vi "Start all.vi"() -> ()   [LabVIEW 2020, in "MeasurementService Editor.lvlib"]
uses:
  _Editor/MeasurementService Editor.lvlib
  0b7fc50c-c44a-4c4b-ba47-f0adf5c9967e.vi
  <vilib>/Comparison/Equal/Equal Functor/Equal Functor.lvclass
panel:
  in  "Run":bool
  in  "Measurement Service":i32[](listbox)
  out "Active Project Name":string
  # "NOTE: This code is depreicated or will not be deployed. The code is maintained so if we need to bring back the \"Start All\" feature, this will be good starting point."
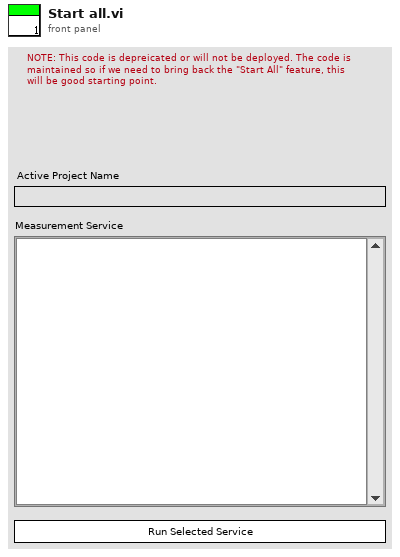
[diagram p1: front panel]
types:
  T1 = cluster{"Project ref":refnum<vi>, "Measurement Service Name":string}
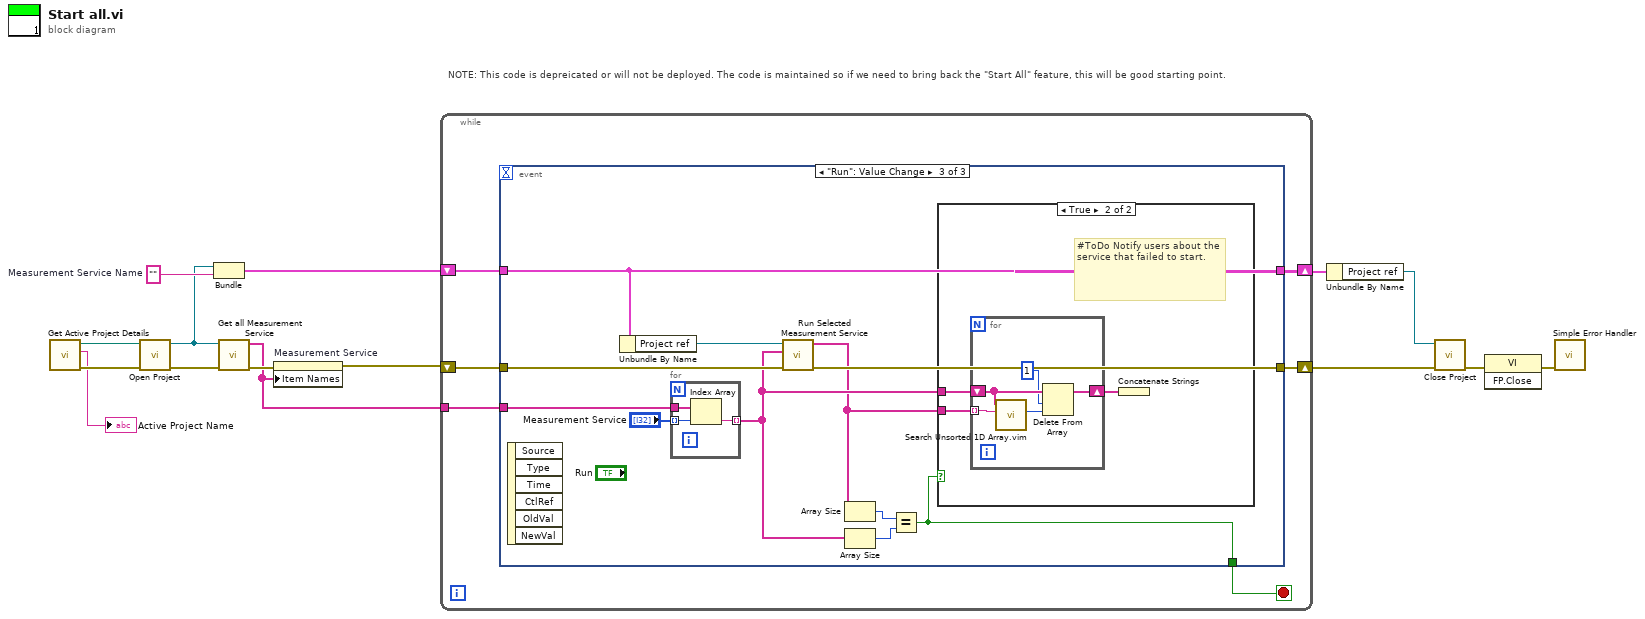
[diagram p0: block diagram]
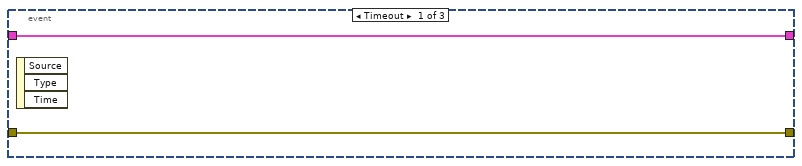
[diagram p2: hidden frame]
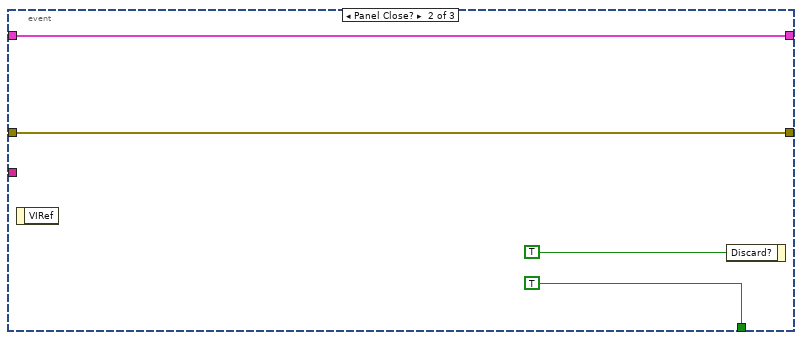
[diagram p3: hidden frame]
diagram:
  w8 = ""  # Measurement Service Name
  # "NOTE: This code is depreicated or will not be deployed. The code is maintained so if we need to bring back the \"Start All\" feature, this will be good starting point."
  n1 = call "Get Active Project Details.vi"() -> ("error out"=w15:errorcluster, "Name"=→"Active Project Name":string, "Path"=w14:path)  [unwired: 9 in]
  n2 = call "Open Project.vi"("error in"=w15, "Path"=w14) -> ("error out"=w5:errorcluster, "Project ref"=w4:refnum<vi>)  [unwired: 8 in]
  n3 = Bundle("Project ref"=w4, "Measurement Service Name"=w8) -> (w12:T1)  [unwired: 1 in]
  n4 = call "Get all Measurement Service.vi"("error in"=w5, "Project ref"=w4) -> ("error out"=w3:errorcluster, "Measurement Service Names"=w1:string[])  [unwired: 8 in]
  n5 = property on="Measurement Service" class="LstBox (strict)"(error in=w3, "Item Names"=w1) -> (error out=w2:errorcluster)  [unwired: 1 in, 1 out]
  n6 = while {
    shift-right: [w20] -> w9
    shift-left: w2 -> [w19]
    shift-right: [w17] -> w11
    shift-left: w12 -> [w18]
    tunnel: w1 -> [w16]
    stop <- w21 stop-if-true
    n7 = event shown="[2] \"Run\": Value Change" {
      selector: _ -> [_ _ _]
      dyn-events: _ -> [_ _ _]
      timeout: _ -> [_ _ _]
      tunnel: [_ TRUE ("Discard?") w31] -> w21
      tunnel: [w23 w25 w30] -> w20
      tunnel: w19 -> [w23 w25 w38]
      tunnel: w18 -> [w22 w24 w37]
      tunnel: [w22 w24 w37] -> w17
      tunnel: w16 -> [_ _ w35]
      event Timeout {
        n8 = event-data() -> ()  [unwired: 1 in, 3 out]
      }
      event Panel Close? {
        n9 = event-data() -> ()  [unwired: 1 in, 1 out]
        n10 = event-data("Discard?"=TRUE) -> ()  [unwired: 1 in, 1 out]
      }
      event "Run": Value Change {
        n11 = event-data() -> ()  [unwired: 1 in, 6 out]
        n12 = Unbundle By Name(w37) -> ("Project ref"=w36:refnum<vi>)
        n13 = for {
          tunnel: w35 -> [w49]
          tunnel: "Measurement Service" -> [w48] mode=indexing
          tunnel: [w47] -> w29 mode=indexing
          n14 = Index Array(array=w49, index=w48) -> (element=w47:string)
        }
        n15 = call "Run Selected Measurement Service.vi"("error in"=w38, "Measurement Service Names"=w29, "Project ref"=w36) -> ("error out"=w30:errorcluster, "Measurement Service Successfully run"=w28:string[])  [unwired: 7 in]
        n16 = Array Size(array=w28) -> (size(s)=w33:i32)
        n17 = Array Size(array=w29) -> (size(s)=w32:i32)
        n18 = Equal?(x=w33, y=w32) -> (x = y?=w31:bool)
        n19 = case shown="True" w31 {
          tunnel: w29 -> [_ w41]
          tunnel: w28 -> [_ w40]
          frame False {
          }
          frame True {
            # "#ToDo Notify users about the service that failed to start."
            n20 = for {
              tunnel: w40 -> [w46] mode=indexing
              shift-right: [w44] -> w39
              shift-left: w41 -> [w45]
              n21 = call "Search Unsorted 1D Array.vim"("element"=w46, "unsorted 1D array"=w45) -> ("index of element"=w43:i32)  [unwired: 9 in]
              n22 = Delete From Array(array=w45, length=1, index=w43) -> (array with subset deleted=w44:string[])  [unwired: 1 out]
            }
            n23 = Concatenate Strings(w39) -> ()  [unwired: 1 out]
          }
        }
      }
    }
  }
  n24 = Unbundle By Name(w11) -> ("Project ref"=w10:refnum<vi>)
  n25 = call "Close Project.vi"("error in"=w9, "Project ref"=w10) -> ("error out"=w7:errorcluster)  [unwired: 9 in]
  n26 = invoke class="VI" method="FP.Close"(error in=w7) -> (error out=w6:errorcluster)  [unwired: 2 in, 2 out]
  n27 = call <vilib>:"Simple Error Handler.vi"("error in (no error)"=w6) -> ()  [unwired: 4 in, 5 out]
